vi "Fetch (Multiple).vi"(4 "Buffer Element2 ()":i32(ring) items=["", "Date", "Extra", "Formatted", "Fractional", "Reading", "Relative", "Seconds", "Status", "Time", "Tstamp", "Unit", "CHAN", "Extra Form", "Extra Unit"], 5 "End Index (10)":i32=10, 6 "Buffer Element1 ()":i32(ring) items=["", "Date", "Extra", "Formatted", "Fractional", "Reading", "Relative", "Seconds", "Status", "Time", "Tstamp", "Unit", "CHAN", "Extra Format", "Extra Unit"], 7 "Start Index (1)":i32=1, 8 "error in (no error)":errorcluster, 9 "Buffer Name (defbuffer1)":string="defbuffer1", 10 "Timeout (100000 ms)":i32=100000, 11 "VISA resource name":refnum<visa-resource-name>) -> (0 "error out":errorcluster, 2 "Measurements":dbl[](array[numeric]), 3 "VISA resource name out":refnum<visa-resource-name>)   [LabVIEW 2020, in "Keithley DMM6500 DAQ6500 Series.lvlib"]
doc: "Reads and returns multiple measurements from the instrument. Use this VI when you want to take multiple measurements using an immediate trigger. Use the low-level VIs for other triggering options."
uses:
  <instrlib>/Keithley DMM6500 DAQ6500 Series/Keithley DMM6500 DAQ6500 Series.lvlib
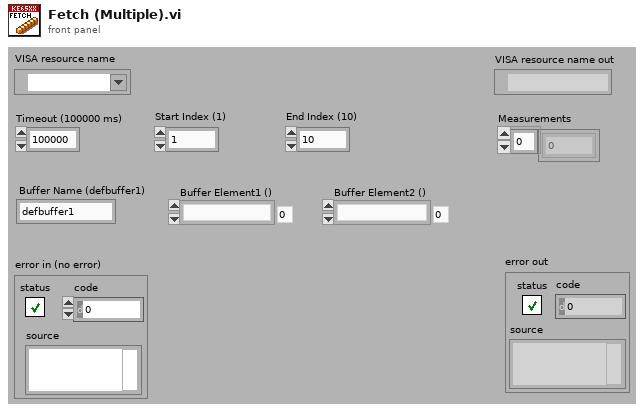
[diagram p1: front panel]
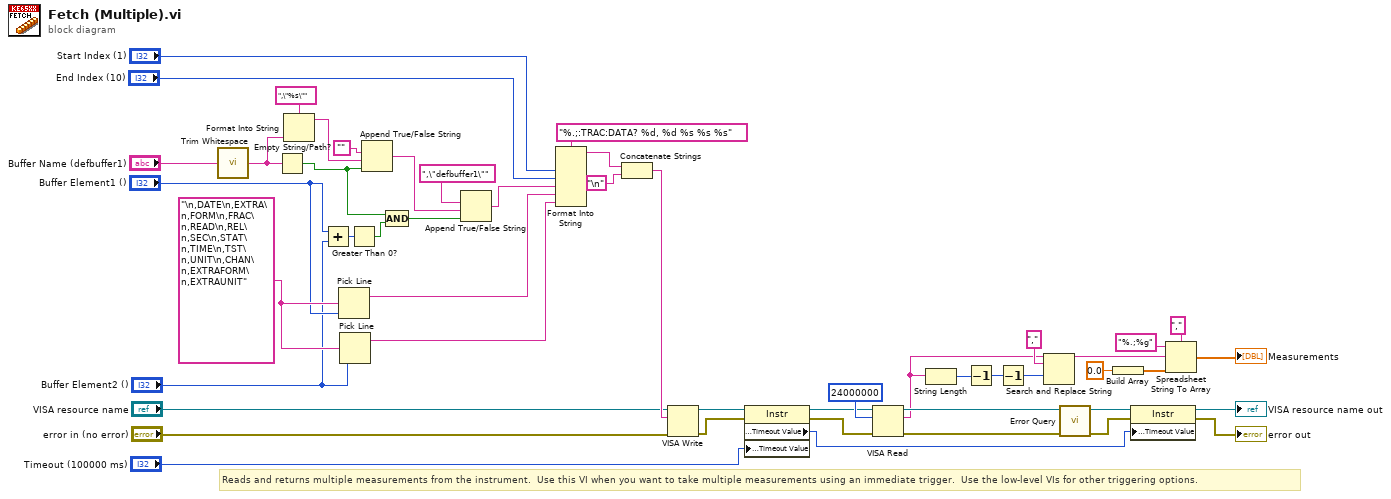
[diagram p0: block diagram]
diagram:
  w12 = "\n,DATE\n,EXTRA\n,FORM\n,FRAC\n,READ\n,REL\n,SEC\n,STAT\n,TIME\n,TST\n,UNIT\n,CHAN\n,EXTRAFORM\n,EXTRAUNIT" ("multi-line string")
  # "Reads and returns multiple measurements from the instrument.  Use this VI when you want to take multiple measurements using an immediate trigger.  Use the low-level VIs for other triggering options."
  n1 = call <vilib>:"Trim Whitespace.vi"("string"="Buffer Name (defbuffer1)") -> ("trimmed string"=w3:string)  [unwired: 1 in]
  n2 = Empty String/Path?(string/path=w3) -> (empty?=w2:bool)
  n3 = Format Into String(format string=",\"%s\"", w3) -> (resulting string=w43:string)  [unwired: 2 in, 1 out]
  n4 = Add(x="Buffer Element1 ()", y="Buffer Element2 ()") -> (x+y=w5:i32)
  n5 = Pick Line(multi-line string=w12, line index="Buffer Element1 ()") -> (output string=w14:string)  [unwired: 1 in]
  n6 = Pick Line(multi-line string=w12, line index="Buffer Element2 ()") -> (output string=w13:string)  [unwired: 1 in]
  n7 = Greater Than 0?(x=w5) -> (x > 0?=w4:bool)
  n8 = Append True/False String(1:w2, 2:w43, 3:"") -> (0:w7:string)  [unwired: 1 in]
  n9 = Compound Arithmetic op=AND(w2, w4) -> (w8:bool)
  n10 = Append True/False String(1:w8, 2:w7, 3:",\"defbuffer1\"" ("true string")) -> (0:w9:string)  [unwired: 1 in]
  n11 = Format Into String(format string="%.;:TRAC:DATA? %d, %d %s %s %s", "Start Index (1)", "End Index (10)", w9, w14, w13) -> (resulting string=w20:string)  [unwired: 2 in, 1 out]
  n12 = Concatenate Strings(w20, "\n") -> (w46:string)
  n13 = VISA Write(VISA resource name="VISA resource name", write buffer=w46, error in (no error)="error in (no error)") -> (VISA resource name out=w30:refnum<visa-resource-name>, error out=w29:errorcluster)  [unwired: 1 out]
  n14 = property on="Property Node" class="Instr"(reference=w30, error in=w29, "General Settings:Timeout Value"="Timeout (100000 ms)") -> (reference out=w27:refnum<visa-resource-name>, error out=w28:errorcluster, "General Settings:Timeout Value"=w22:u32)
  n15 = VISA Read(VISA resource name=w27, byte count=i64 24000000, error in (no error)=w28) -> (VISA resource name out=w48:refnum<visa-resource-name>, read buffer=w32:string, error out=w47:errorcluster)  [unwired: 1 out]
  n16 = String Length(string=w32) -> (length=w35:i32)
  n17 = Decrement(x=w35) -> (x-1=w33:i32)
  n18 = Decrement(x=w33) -> (x-1=w34:i32)
  n19 = Search and Replace String(input string=w32, search string=",", offset=w34) -> (result string=w38:string)  [unwired: 5 in, 3 out]
  n20 = call <instrlib>:"Error Query.vi"("error in (no error)"=w47, "VISA resource name"=w48) -> ("error out"=w24:errorcluster, "VISA resource name out"=w26:refnum<visa-resource-name>)  [unwired: 6 in, 2 out]
  n21 = Build Array(0.0 ("element")) -> (w41:dbl[])
  n22 = property on="Property Node" class="Instr"(reference=w26, error in=w24, "General Settings:Timeout Value"=w22) -> (reference out=→"VISA resource name out":refnum<visa-resource-name>, error out=→"error out":errorcluster)
  n23 = Spreadsheet String To Array(delimiter (Tab)=",", format string="%.;%g", spreadsheet string=w38, array type (2D Dbl)=w41) -> (array=→"Measurements":dbl[])
